vi "user32_SetForegroundWindow.vi"(8 "error in (no error)":errorcluster, 11 "hwnd":i64) -> (0 "error out":errorcluster, 3 "Return":i32)   [LabVIEW 2020]
uses:
  user32.dll
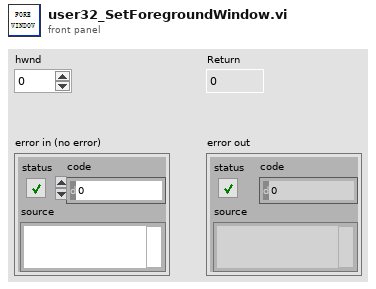
[diagram p1: front panel]
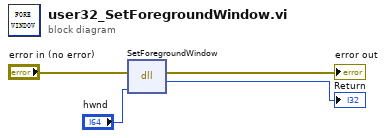
[diagram p0: block diagram]
diagram:
  n1 = dll-call lib="user32.dll" fn="SetForegroundWindow"(error in="error in (no error)", "hwnd"="hwnd") -> (error out=→"error out":errorcluster, "返回值"=→"Return":i32)  [unwired: 3 in, 1 out]
